vi "USB2XXX_LINEX_SlaveTest.vi"() -> ()   [LabVIEW 2010]
panel:
  out "从机读取到的数据帧数":i32
  in  "pInMsg 3":T1={"Timestamp"=20, "MsgType"=3, "CheckType"=1, "DataLen"=8, "Sync"=85, "PID"=3, "Data[0]"=33, "Data[1]"=34, "Data[2]"=35, "Data[3]"=36, "Data[4]"=37, "Data[5]"=38, "Data[6]"=39, "Data[7]"=40, "Check"=1, "Reserve"=0, "Reserve"=0} {"Sync" format="%x"; "PID" format="%x"; "Data[0]" format="%x"; "Data[1]" format="%x"; "Data[2]" format="%x"; "Data[3]" format="%x"; "Data[4]" format="%x"; "Data[5]" format="%x"; "Data[6]" format="%x"; "Data[7]" format="%x"; "Check" format="%x"; "Reserve" format="%x"; "Reserve" format="%x"}
  in  "pInMsg 2":T1={"Timestamp"=20, "MsgType"=3, "CheckType"=1, "DataLen"=8, "Sync"=85, "PID"=2, "Data[0]"=17, "Data[1]"=18, "Data[2]"=19, "Data[3]"=20, "Data[4]"=21, "Data[5]"=22, "Data[6]"=23, "Data[7]"=24, "Check"=1, "Reserve"=0, "Reserve"=0} {"Sync" format="%x"; "PID" format="%x"; "Data[0]" format="%x"; "Data[1]" format="%x"; "Data[2]" format="%x"; "Data[3]" format="%x"; "Data[4]" format="%x"; "Data[5]" format="%x"; "Data[6]" format="%x"; "Data[7]" format="%x"; "Check" format="%x"; "Reserve" format="%x"; "Reserve" format="%x"}
  out "pOutMsg":T2(array[cluster]) {"Sync" format="%x"; "PID" format="%x"; "Data[0]" format="%x"; "Data[1]" format="%x"; "Data[2]" format="%x"; "Data[3]" format="%x"; "Data[4]" format="%x"; "Data[5]" format="%x"; "Data[6]" format="%x"; "Data[7]" format="%x"; "Check" format="%x"}
  in  "pInMsg":T1={"Timestamp"=20, "MsgType"=3, "CheckType"=1, "DataLen"=8, "Sync"=85, "PID"=1, "Data[0]"=1, "Data[1]"=2, "Data[2]"=3, "Data[3]"=4, "Data[4]"=5, "Data[5]"=6, "Data[6]"=7, "Data[7]"=8, "Check"=1, "Reserve"=0, "Reserve"=0} {"Sync" format="%x"; "PID" format="%x"; "Data[0]" format="%x"; "Data[1]" format="%x"; "Data[2]" format="%x"; "Data[3]" format="%x"; "Data[4]" format="%x"; "Data[5]" format="%x"; "Data[6]" format="%x"; "Data[7]" format="%x"; "Check" format="%x"; "Reserve" format="%x"; "Reserve" format="%x"}
  out "function return":i32
  in  "BaudRate":u32=19200
  in  "Channel Index":u8(ring) items=["CH0"]
  in  "Device Index":i32(ring) items=["0", "1", "2", "3", "4", "5"]
  out "Flag(T:Write;F:Read)":bool=TRUE
  in  "stop":bool
  in  "Read":bool
  in  "Write":bool
  # "波特率一定要设置，否则程序可能出错"
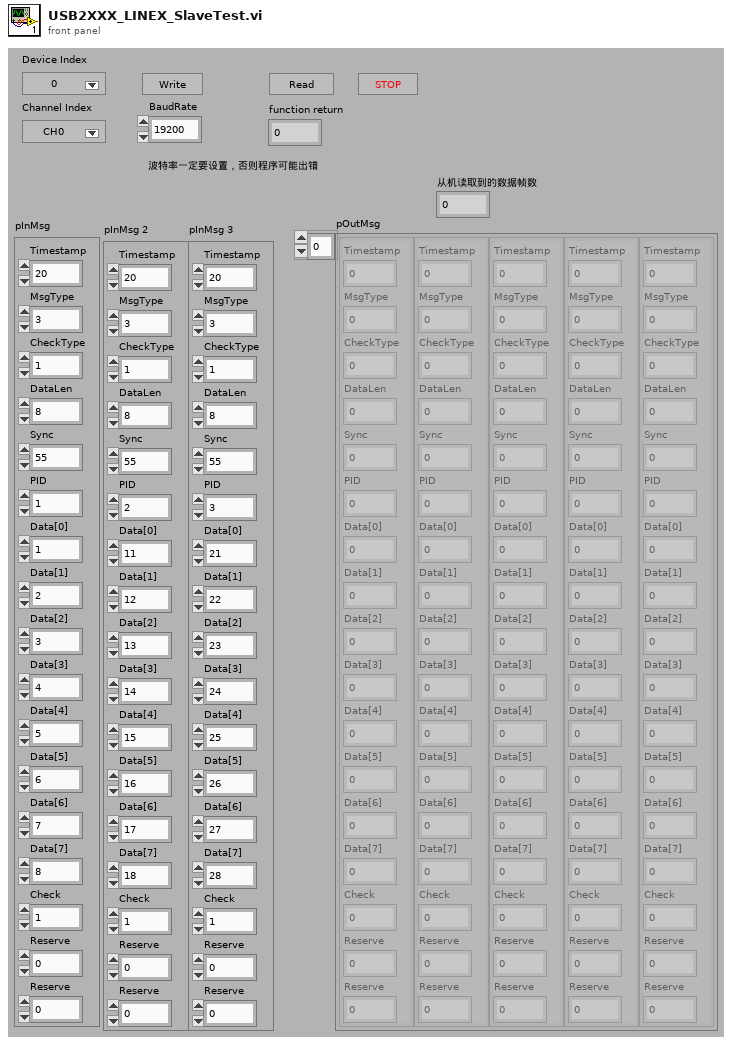
[diagram p1: front panel]
types:
  T1 = cluster{"Timestamp":u32, "MsgType":u8, "CheckType":u8, "DataLen":u8, "Sync":u8, "PID":u8, "Data[0]":u8, "Data[1]":u8, "Data[2]":u8, "Data[3]":u8, "Data[4]":u8, "Data[5]":u8, "Data[6]":u8, "Data[7]":u8, "Check":u8, "Reserve":u8, "Reserve":u8}
  T2 = cluster{"Timestamp":u32, "MsgType":u8, "CheckType":u8, "DataLen":u8, "Sync":u8, "PID":u8, "Data[0]":u8, "Data[1]":u8, "Data[2]":u8, "Data[3]":u8, "Data[4]":u8, "Data[5]":u8, "Data[6]":u8, "Data[7]":u8, "Check":u8, "Reserve":u8, "Reserve":u8}[]
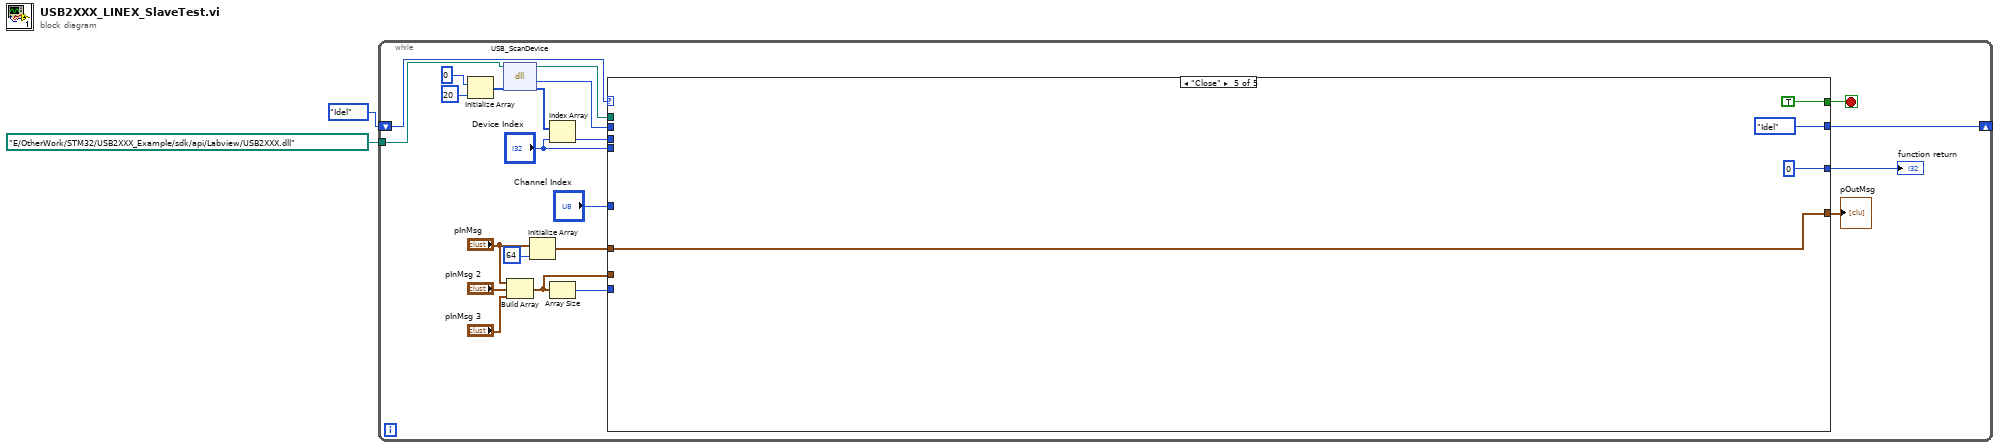
[diagram p0: block diagram]
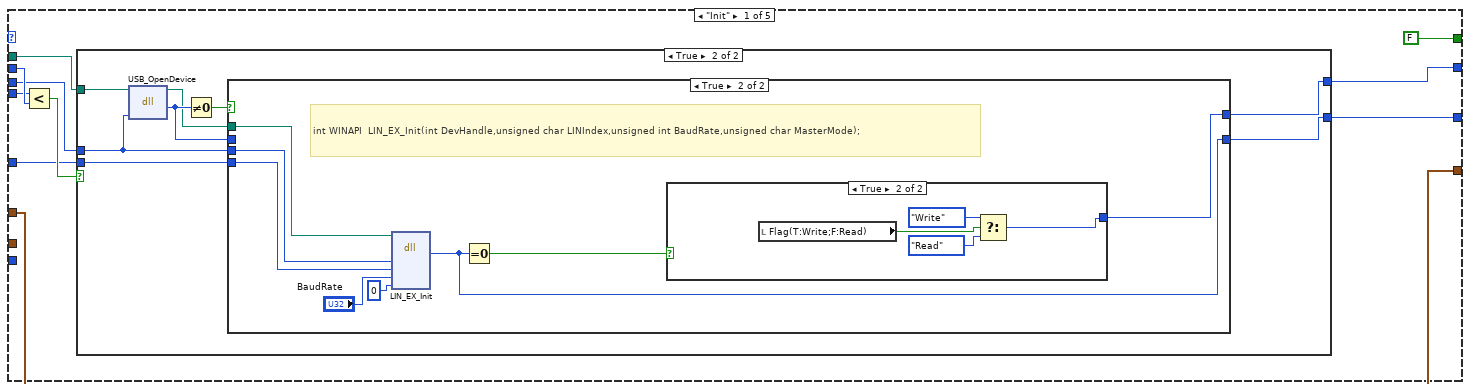
[diagram p2: hidden frame]
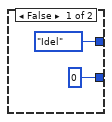
[diagram p3: hidden frame]
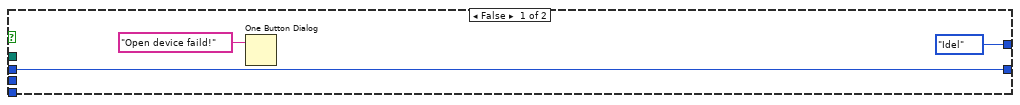
[diagram p4: hidden frame]
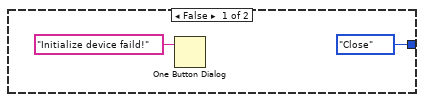
[diagram p5: hidden frame]
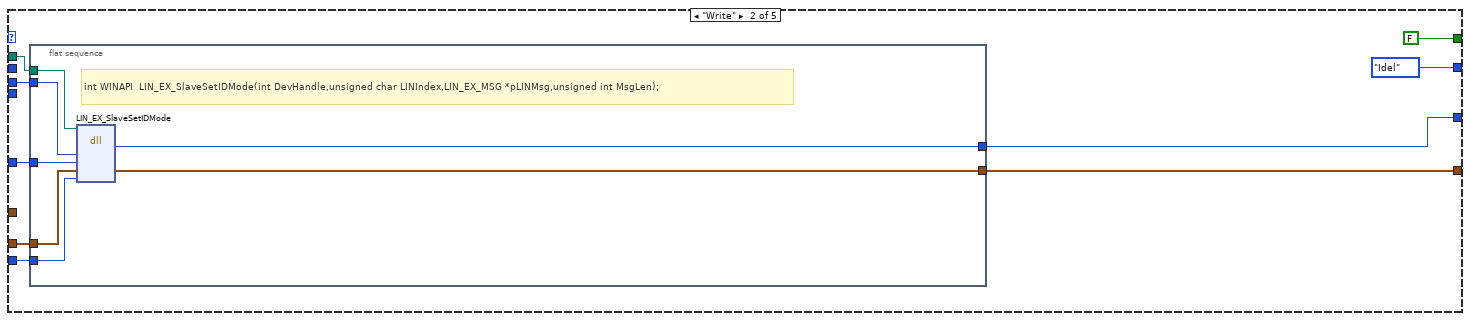
[diagram p6: hidden frame]
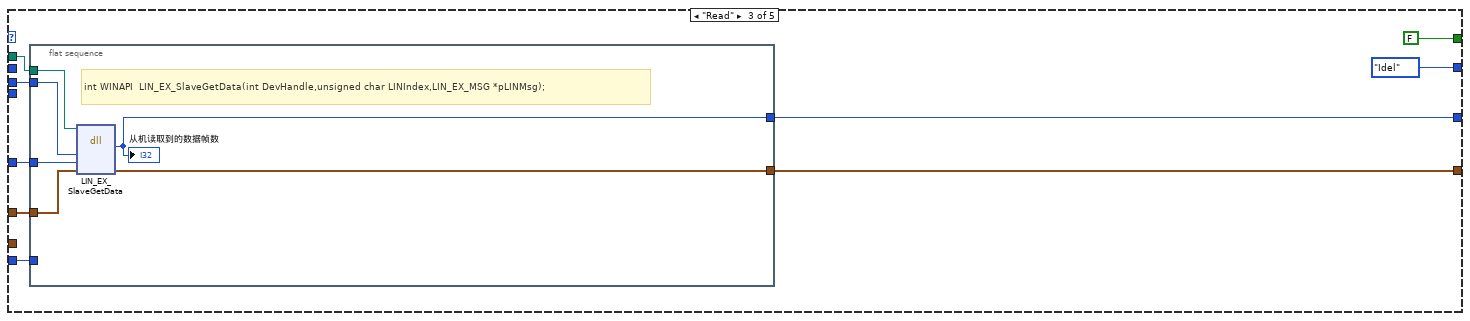
[diagram p7: hidden frame]
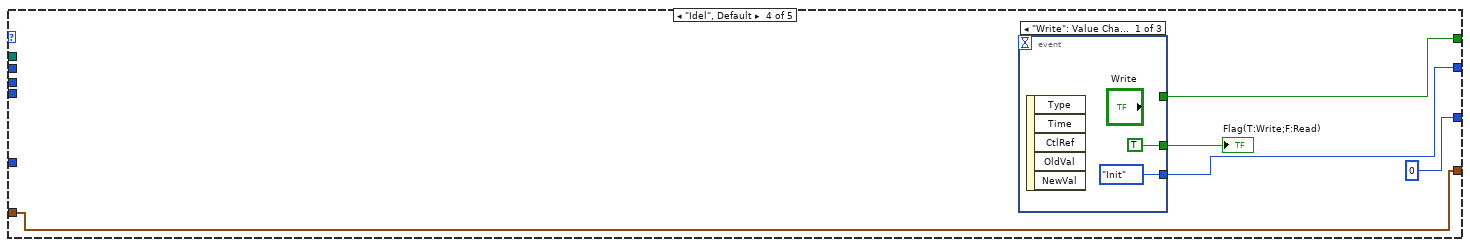
[diagram p8: hidden frame]
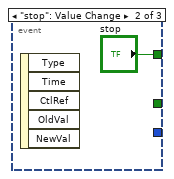
[diagram p9: hidden frame]
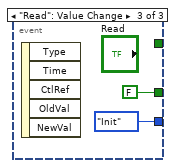
[diagram p10: hidden frame]
diagram:
  n1 = while {
    shift-right: [w23] -> _
    shift-left: enum16{"Init", "Write", "Read", "Idel", "Close"}."Idel" ("Enum") -> [w24]
    tunnel: path "E:/OtherWork/STM32/USB2XXX_Example/sdk/api/Labview/USB2XXX.dll" ("path in") -> [w4]
    stop <- w21 stop-if-true
    n2 = Initialize Array(0, 20 ("dimension size")) -> (w20:i32[])
    n3 = dll-call lib="E:/OtherWork/STM32/USB2XXX_Example/trunk/Labview/PublicFiles/USB2XXX.dll" fn="USB_ScanDevice"(path in=w4, "pDevNum"=w20) -> (path out=w3:path, "return type"=w16:i32, "pDevNum"=w17:i32[])  [unwired: 2 in, 1 out]
    n4 = Build Array("pInMsg", "pInMsg 2", "pInMsg 3") -> (w9:T2)
    n5 = Initialize Array("pInMsg", 64 ("dimension size")) -> (w5:T2)
    n6 = Index Array(array=w17, index="Device Index") -> (element=w12:i32)
    n7 = Array Size(array=w9) -> (size(s)=w8:i32)
    n8 = case shown="\"Close\"" w24 {
      tunnel: [w33 enum16{"Init", "Write", "Read", "Idel", "Close"}."Idel" ("Enum") enum16{"Init", "Write", "Read", "Idel", "Close"}."Idel" ("Enum") w95 enum16{"Init", "Write", "Read", "Idel", "Close"}."Idel" ("Enum")] -> w23
      tunnel: w12 -> [w29 w67 w84 _ _]
      tunnel: "Channel Index" -> [w32 w66 w83 _ _]
      tunnel: [FALSE FALSE FALSE w96 TRUE] -> w21
      tunnel: w16 -> [w30 _ _ _ _]
      tunnel: "Device Index" -> [w28 _ _ _ _]
      tunnel: w8 -> [_ w63 w81 _ _]
      tunnel: w5 -> [w27 _ w82 w94 w104]
      tunnel: w9 -> [_ w68 _ _ _]
      tunnel: [w27 w65 w79 w94 w104] -> w14
      tunnel: [w26 w64 w80 0 ("return type") 0 ("return type")] -> w13
      tunnel: w3 -> [w25 w62 w78 _ _]
      frame "Init" {
        n9 = Less?(x=w28, y=w30) -> (x < y?=w34:bool)
        n10 = case shown="True" w34 {
          tunnel: w29 -> [_ w42]
          tunnel: w32 -> [_ w43]
          tunnel: [enum16{"Init", "Write", "Read", "Idel", "Close"}."Idel" ("Enum") w41] -> w33
          tunnel: [0 ("return type") w40] -> w26
          tunnel: w25 -> [_ w38]
          frame False {
          }
          frame True {
            n11 = dll-call lib="E:/OtherWork/STM32/USB2XXX_Example/trunk/Labview/PublicFiles/USB2XXX.dll" fn="USB_OpenDevice"(path in=w38, "DevIndex"=w42) -> (path out=w37:path, "return type"=w39:u8)  [unwired: 3 in, 1 out]
            n12 = Not Equal To 0?(x=w39) -> (x != 0?=w44:bool)
            n13 = case shown="True" w44 {
              tunnel: w43 -> [_ w51]
              tunnel: w42 -> [_ w52]
              tunnel: [enum16{"Init", "Write", "Read", "Idel", "Close"}."Idel" ("Enum") w54] -> w41
              tunnel: [w45 w49] -> w40
              tunnel: w39 -> [w45 _]
              tunnel: w37 -> [_ w48]
              frame False {
                n14 = One Button Dialog(message="Open device faild!") -> ()  [unwired: 1 in, 1 out]
              }
              frame True {
                # "int WINAPI  LIN_EX_Init(int DevHandle,unsigned char LINIndex,unsigned int BaudRate,unsigned char MasterMode);"
                n15 = dll-call lib="E:/OtherWork/STM32/USB2XXX_Example/trunk/Labview/PublicFiles/USB2XXX.dll" fn="LIN_EX_Init"(path in=w48, "DevHandle"=w52, "LINIndex"=w51, "BaudRate"="BaudRate", "MasterMode"=u8 0) -> ("return type"=w49:i32)  [unwired: 6 in, 2 out]
                n16 = Equal To 0?(x=w49) -> (x = 0?=w55:bool)
                n17 = case shown="True" w55 {
                  tunnel: [enum16{"Init", "Write", "Read", "Idel", "Close"}."Close" ("Enum") w58] -> w54
                  frame False {
                    n18 = One Button Dialog(message="Initialize device faild!") -> ()  [unwired: 1 in, 1 out]
                  }
                  frame True {
                    n19 = local read "Flag(T:Write;F:Read)"() -> (w61:bool)
                    n20 = Select(t=enum16{"Init", "Write", "Read", "Idel", "Close"}."Write" ("Enum"), s=w61, f=enum16{"Init", "Write", "Read", "Idel", "Close"}."Read" ("Enum")) -> (s? t:f=w58:enum16{"Init", "Write", "Read", "Idel", "Close"})
                  }
                }
              }
            }
          }
        }
      }
      frame "Write" {
        n21 = flat-sequence {
          tunnel: w67 -> [w76]
          tunnel: w66 -> [w75]
          tunnel: [w77] -> w65
          tunnel: [w72] -> w64
          tunnel: w63 -> [w73]
          tunnel: w68 -> [w74]
          tunnel: w62 -> [w71]
          frame #0 {
            # "int WINAPI  LIN_EX_SlaveSetIDMode(int DevHandle,unsigned char LINIndex,LIN_EX_MSG *pLINMsg,unsigned int MsgLen);"
            n22 = dll-call lib="E:/OtherWork/STM32/USB2XXX_Example/trunk/Labview/PublicFiles/USB2XXX.*" fn="LIN_EX_SlaveSetIDMode"(path in=w71, "DevHandle"=w76, "LINIndex"=w75, "pLINMsg"=w74, "MsgLen"=w73) -> ("return type"=w72:i32, "pLINMsg"=w77:T2)  [unwired: 5 in, 2 out]
          }
        }
      }
      frame "Read" {
        n23 = flat-sequence {
          tunnel: w84 -> [w92]
          tunnel: w83 -> [w91]
          tunnel: w82 -> [w90]
          tunnel: [w88] -> w80
          tunnel: [w89] -> w79
          tunnel: w81 -> [_]
          tunnel: w78 -> [w87]
          frame #0 {
            # "int WINAPI  LIN_EX_SlaveGetData(int DevHandle,unsigned char LINIndex,LIN_EX_MSG *pLINMsg);"
            n24 = dll-call lib="E:/OtherWork/STM32/USB2XXX_Example/trunk/Labview/PublicFiles/USB2XXX.*" fn="LIN_EX_SlaveGetData"(path in=w87, "DevHandle"=w92, "LINIndex"=w91, "pLINMsg"=w90) -> ("return type"=w88:i32, "pLINMsg"=w89:T2)  [unwired: 4 in, 2 out]
            "从机读取到的数据帧数" <- w88
          }
        }
      }
      frame "Idel", Default {
        n25 = event shown="[0] \"Write\": Value Change" {
          selector: _ -> [_ _ _]
          dyn-events: _ -> [_ _ _]
          timeout: _ -> [_ _ _]
          tunnel: [TRUE _ FALSE] -> w97
          tunnel: [_ "stop" _] -> w96
          tunnel: [enum16{"Init", "Write", "Read", "Idel", "Close"}."Init" ("Enum") _ enum16{"Init", "Write", "Read", "Idel", "Close"}."Init" ("Enum")] -> w95
          event "Write": Value Change {
            n26 = event-data() -> ()  [unwired: 1 in, 5 out]
          }
          event "stop": Value Change {
            n27 = event-data() -> ()  [unwired: 1 in, 5 out]
          }
          event "Read": Value Change {
            n28 = event-data() -> ()  [unwired: 1 in, 5 out]
          }
        }
        "Flag(T:Write;F:Read)" <- w97
      }
      frame "Close" {
      }
    }
    "pOutMsg" <- w14
    "function return" <- w13
  }
